vi "Up_2PatternMatch.vi"(6 "error in":errorcluster, 8 "Set":bool=TRUE, 9 "Image Dst In":T2, 10 "ROI2":string, 11 "ROI1":string) -> (0 "TestResult1 2":T1 {"Angl" format="%#_13g"}, 1 "Result":string, 2 "TestResult1":T1 {"Angl" format="%#_13g"}, 3 "Refnum out":T2(plugin-control), 4 "error out":errorcluster)   [LabVIEW 2019]
uses:
  <vilib>/vision/Image Controls.llb/IMAQ Image.ctl
  Ctrl/UpGrayImg.ctl
  Ctrl/UpColorImg.ctl
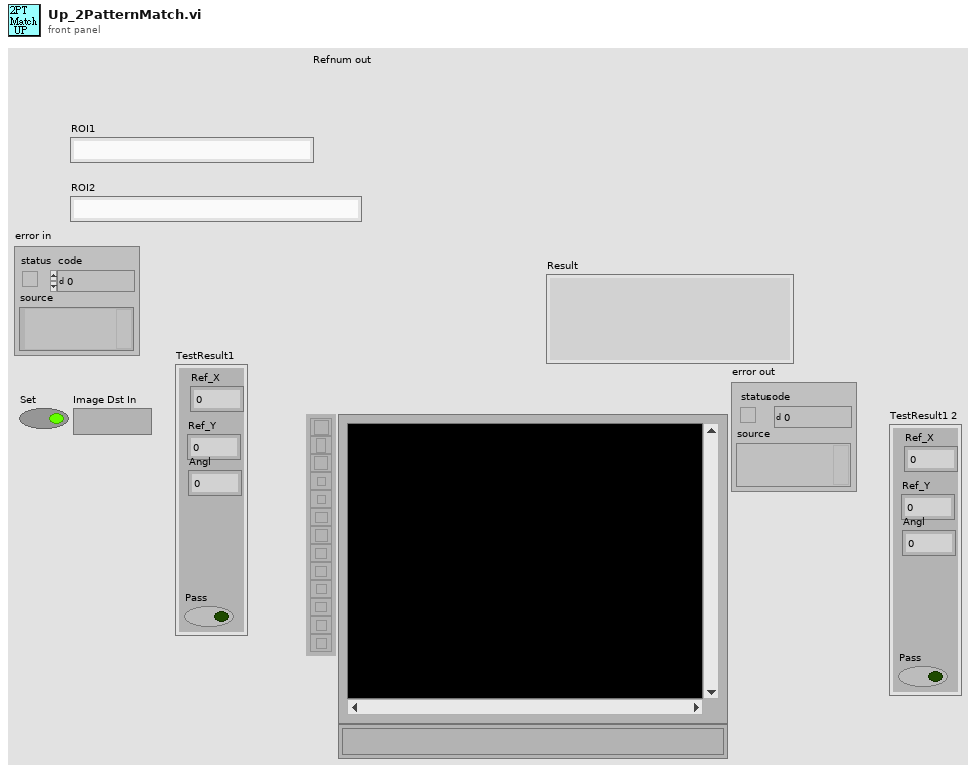
[diagram p1: front panel]
types:
  T1 = cluster{"Ref_X":dbl, "Ref_Y":dbl, "Angl":dbl, "Pass":bool}
  T2 = typedef "IMAQ Image.ctl" = refnum<image>
  T3 = cluster{"X":dbl, "X 2":dbl, "Angl":dbl, "Pass":bool}
  T4 = typedef "UpColorImg.ctl" = enum16{"CUpCam", "CUpSource", "CUpShow", "CUpToProcess1", "CUpToProcess2", "CUpForMatch", "CUpForCheckNumbers", "CupPreProcess"}
  T5 = typedef "UpGrayImg.ctl" = enum16{"CUpGray", "CUpProce1", "CUpProce2", "UpPattern1", "UpPattern2", "UpCalibImg", "UpPreProcess"}
  T6 = cluster{"Position":cluster{"x":sgl, "y":sgl}, "Angle":sgl, "Score":sgl}
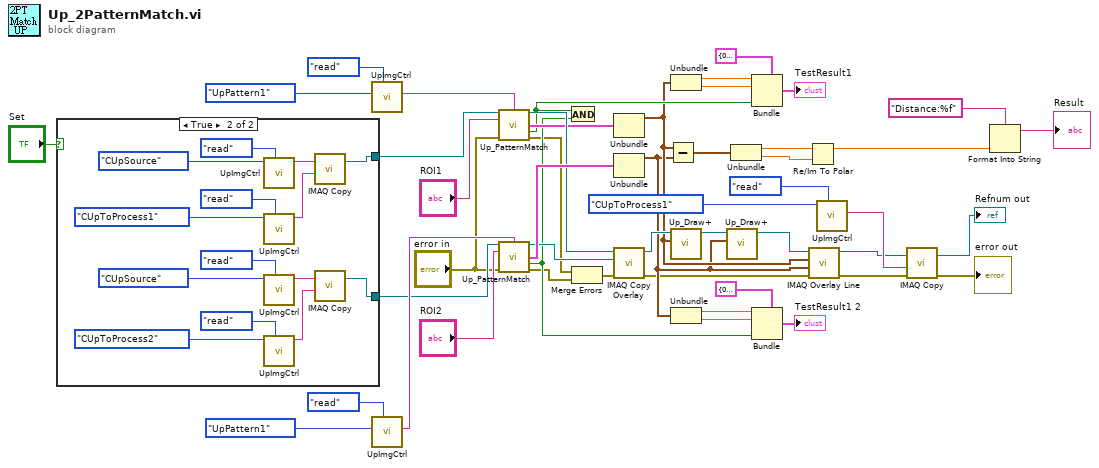
[diagram p0: block diagram]
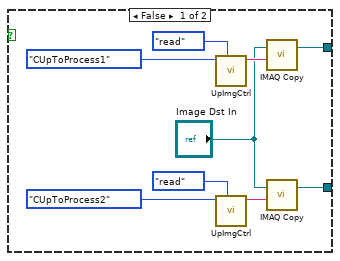
[diagram p2: hidden frame]
diagram:
  n1 = case shown="True" "Set" {
    tunnel: [w49 w58] -> w9
    tunnel: [w54 w59] -> w8
    frame False {
      n2 = call "UpImgCtrl.vi"("Action"=enum16{"Initial", "read", "release"}."read", "ColorImg 2"=UpColorImg."CUpToProcess1") -> ("ColorImg"=w53:string)  [unwired: 8 in, 1 out]
      n3 = call "UpImgCtrl.vi"("Action"=enum16{"Initial", "read", "release"}."read", "ColorImg 2"=UpColorImg."CUpToProcess2") -> ("ColorImg"=w55:string)  [unwired: 8 in, 1 out]
      n4 = call "IMAQ Copy"("Image Dst"=w53, "Image Src"="Image Dst In") -> ("Image Dst Out"=w49:T2)  [unwired: 4 in, 1 out]
      n5 = call "IMAQ Copy"("Image Dst"=w55, "Image Src"="Image Dst In") -> ("Image Dst Out"=w54:T2)  [unwired: 4 in, 1 out]
    }
    frame True {
      n6 = call "UpImgCtrl.vi"("Action"=enum16{"Initial", "read", "release"}."read", "ColorImg 2"=UpColorImg."CUpSource") -> ("ColorImg"=w69:string)  [unwired: 8 in, 1 out]
      n7 = call "UpImgCtrl.vi"("Action"=enum16{"Initial", "read", "release"}."read", "ColorImg 2"=UpColorImg."CUpToProcess1") -> ("ColorImg"=w71:string)  [unwired: 8 in, 1 out]
      n8 = call "UpImgCtrl.vi"("Action"=enum16{"Initial", "read", "release"}."read", "ColorImg 2"=UpColorImg."CUpSource") -> ("ColorImg"=w61:string)  [unwired: 8 in, 1 out]
      n9 = call "UpImgCtrl.vi"("Action"=enum16{"Initial", "read", "release"}."read", "ColorImg 2"=UpColorImg."CUpToProcess2") -> ("ColorImg"=w60:string)  [unwired: 8 in, 1 out]
      n10 = call "IMAQ Copy"("Image Dst"=w71, "Image Src"=w69) -> ("Image Dst Out"=w58:T2)  [unwired: 4 in, 1 out]
      n11 = call "IMAQ Copy"("Image Dst"=w60, "Image Src"=w61) -> ("Image Dst Out"=w59:T2)  [unwired: 4 in, 1 out]
    }
  }
  n12 = call "UpImgCtrl.vi"("Action"=enum16{"Initial", "read", "release"}."read", "GrayImg 2"=UpGrayImg."UpPattern1") -> ("GrayImg"=w25:string)  [unwired: 8 in, 1 out]
  n13 = call "UpImgCtrl.vi"("Action"=enum16{"Initial", "read", "release"}."read", "GrayImg 2"=UpGrayImg."UpPattern1") -> ("GrayImg"=w36:string)  [unwired: 8 in, 1 out]
  n14 = call "Up_PatternMatch.vi"("Image In"=w9, "Template Image"=w25, "ROIIn"="ROI1", "error in"="error in") -> ("Image Out"=w41:T2, "ResultShow"=w24:T6, "OK"=w23:bool, "error out"=w7:errorcluster)  [unwired: 5 in, 3 out]
  n15 = call "Up_PatternMatch.vi"("Image In"=w8, "Template Image"=w36, "ROIIn"="ROI2", "error in"="error in") -> ("Image Out"=w42:T2, "ResultShow"=w48:T6, "OK"=w20:bool, "error out"=w6:errorcluster)  [unwired: 5 in, 3 out]
  n16 = And(x=w23, y=w20) -> ()  [unwired: 1 out]
  n17 = Merge Errors(w7, w6) -> (w5:errorcluster)
  n18 = Unbundle(w24) -> ("Position"=w15:cluster{"x":sgl, "y":sgl})  [unwired: 2 out]
  n19 = Unbundle(w48) -> ("Position"=w14:cluster{"x":sgl, "y":sgl})  [unwired: 2 out]
  n20 = call "IMAQ Copy Overlay"("error in (no error)"=w5, "Image Dst"=w42, "Image Src"=w41) -> ("error out"=w4:errorcluster, "Image Dst Out"=w34:T2)  [unwired: 7 in]
  n21 = Subtract(x=w15, y=w14) -> (x-y=w13:cluster{"x":sgl, "y":sgl})
  n22 = Unbundle(w15) -> ("x"=w19:sgl, "y"=w18:sgl)
  n23 = call "Up_Draw+.vi"("Center"=w15, "Image"=w34) -> ("Image Out"=w30:T2)  [unwired: 9 in]
  n24 = Unbundle(w14) -> ("x"=w17:sgl, "y"=w16:sgl)
  n25 = call "Up_Draw+.vi"("Center"=w14, "Image"=w30) -> ("Image Out"=w27:T2)  [unwired: 9 in]
  n26 = Unbundle(w13) -> ("x"=w12:sgl, "y"=w11:sgl)
  n27 = Bundle(cluster=T3 {"X"=0.0, "X 2"=0.0, "Angl"=0.0, "Pass"=FALSE} ("TestResult"), "X"=w19, "X 2"=w18, "Pass"=w23) -> (→"TestResult1":T3)  [unwired: 1 in]
  n28 = Bundle(cluster=T3 {"X"=0.0, "X 2"=0.0, "Angl"=0.0, "Pass"=FALSE} ("TestResult"), "X"=w17, "X 2"=w16, "Pass"=w20) -> (→"TestResult1 2":T3)  [unwired: 1 in]
  n29 = Re/Im To Polar(2:w11, 3:w12) -> (1:w10:sgl)  [unwired: 1 out]
  n30 = call "IMAQ Overlay Line"("error in (no error)"=w4, "End Point"=w14, "Start Point"=w15, "Image"=w27) -> ("error out"=w3:errorcluster, "Image Out"=w26:T2)  [unwired: 6 in]
  n31 = call "UpImgCtrl.vi"("Action"=enum16{"Initial", "read", "release"}."read", "ColorImg 2"=UpColorImg."CUpToProcess1") -> ("GrayImg"=w45:string)  [unwired: 8 in, 1 out]
  n32 = call "IMAQ Copy"("error in (no error)"=w3, "Image Dst"=w45, "Image Src"=w26) -> ("error out"=→"error out":errorcluster, "Image Dst Out"=→"Refnum out":T2)  [unwired: 3 in]
  n33 = Format Into String(format string="Distance:%f", w10) -> (resulting string=→"Result":string)  [unwired: 2 in, 1 out]
